vi "UI Build Holding Reg CMD.vi"(8 "error in (no error)":errorcluster, 9 "Message Data":variant, 11 "DAQ DO ON-OFF":refnum<queue>) -> (0 "error out":errorcluster, 1 "CMD Data":variant, 3 "CMD Queue out":refnum<queue>)   [LabVIEW 2020]
uses:
  support/Message Queue/Message Cluster.ctl
  support/Message Queue/Message Queue.lvlib
panel:
  in  "Register":T1(ring)
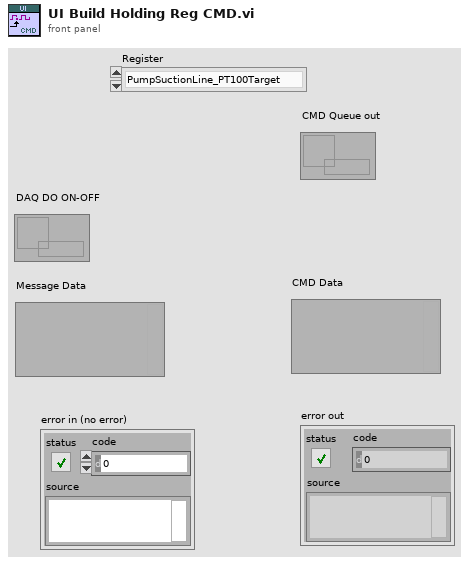
[diagram p1: front panel]
types:
  T1 = enum16{"PumpSuctionLine_PT100Target", "PumpSuctionLine_PT100LimitMin", "PumpSuctionLine_PT100LimitMax", "PumpMainLine_PressureTarget", "PumpMainLine_PressureTargetMin", "PumpMainLine_PressureTargetMax", "RPMTarget", "RPMTargetMax", "RPMTargetMin", "PumpSuctionLine_PressureTarget", "PumpSuctionLine_PressureTargetMin", "PumpSuctionLine_PressureTargetMax", "PumpMainLine_MaxPressureLimit", "PumpSuctionLine_MaxPressureLimit", "PumpSuctionLine_MinPressureLimit", "PumpDrainLine_MaxPressureLimit", "PumpReplenishmentLine_MinPressureLimit", "DrainMinusSuctionPressureLimit", "Torque_MaxLimit", "SectorNumber", "RowNumber", "ProcedureNumber", "ResetControl", "DigitalControl", "CommNumber", "ProcessTimerTarget"}
  T2 = cluster{"Register":enum16{"PumpSuctionLine_PT100Target", "PumpSuctionLine_PT100LimitMin", "PumpSuctionLine_PT100LimitMax", "PumpMainLine_PressureTarget", "PumpMainLine_PressureTargetMin", "PumpMainLine_PressureTargetMax", "RPMTarget", "RPMTargetMax", "RPMTargetMin", "PumpSuctionLine_PressureTarget", "PumpSuctionLine_PressureTargetMin", "PumpSuctionLine_PressureTargetMax", "PumpMainLine_MaxPressureLimit", "PumpSuctionLine_MaxPressureLimit", "PumpSuctionLine_MinPressureLimit", "PumpDrainLine_MaxPressureLimit", "PumpReplenishmentLine_MinPressureLimit", "DrainMinusSuctionPressureLimit", "Torque_MaxLimit", "SectorNumber", "RowNumber", "ProcedureNumber", "ResetControl", "DigitalControl", "CommNumber", "ProcessTimerTarget"}, "value":u16}
  T3 = typedef "Test Names.ctl" = u16
  T4 = cluster{"Register":enum16{"PumpSuctionLine_PT100Target", "PumpSuctionLine_PT100LimitMin", "PumpSuctionLine_PT100LimitMax", "PumpMainLine_PressureTarget", "PumpMainLine_PressureTargetMin", "PumpMainLine_PressureTargetMax", "RPMTarget", "RPMTargetMax", "RPMTargetMin", "PumpSuctionLine_PressureTarget", "PumpSuctionLine_PressureTargetMin", "PumpSuctionLine_PressureTargetMax", "PumpMainLine_MaxPressureLimit", "PumpSuctionLine_MaxPressureLimit", "PumpSuctionLine_MinPressureLimit", "PumpDrainLine_MaxPressureLimit", "PumpReplenishmentLine_MinPressureLimit", "DrainMinusSuctionPressureLimit", "Torque_MaxLimit", "SectorNumber", "RowNumber", "ProcedureNumber", "ResetControl", "DigitalControl", "CommNumber", "ProcessTimerTarget"}, "value":u16}[]
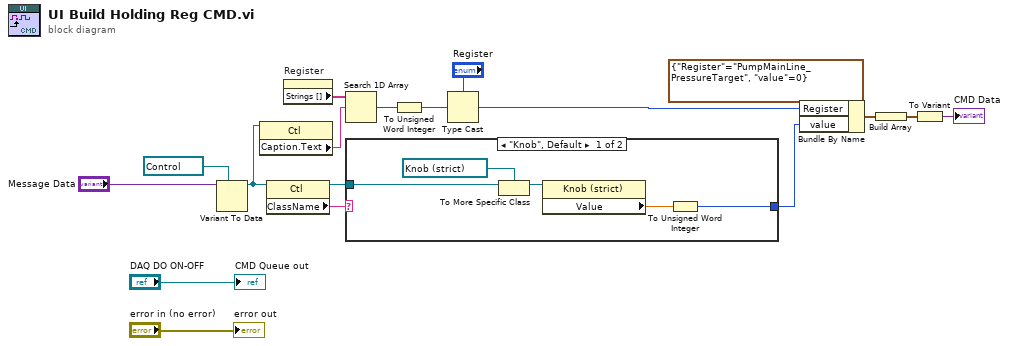
[diagram p0: block diagram]
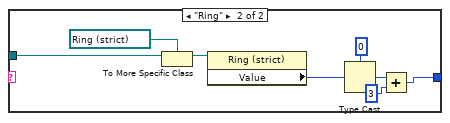
[diagram p2: hidden frame]
diagram:
  n1 = Variant To Data(type=refnum<vi> refnum ("CtlRef"), Variant="Message Data") -> (data=w2:refnum<vi>)  [unwired: 1 in, 1 out]
  n2 = property class="Ctl"(reference=w2) -> ("Caption.Text"=w14:string)  [unwired: 1 in, 2 out]
  n3 = property class="Ctl"(reference=w2) -> (reference out=w3:refnum<vi>, "ClassName"=w4:string)  [unwired: 1 in, 1 out]
  n4 = property on="Register" class="Enum (strict)"() -> ("Strings []"=w13:string[])  [unwired: 2 in, 2 out]
  n5 = Search 1D Array(1D array=w13, element=w14) -> (index of element=w11:i32)  [unwired: 1 in]
  n6 = case shown="\"Knob\", Default" w4 {
    tunnel: w3 -> [w23 w31]
    tunnel: [w19 w25] -> w1
    frame "Knob", Default {
      n7 = To More Specific Class(target class=refnum<vi> refnum ("Manual Air Pressure Control"), reference=w23) -> (specific class reference=w21:refnum<vi>)  [unwired: 1 in, 1 out]
      n8 = property class="Knob (strict)"(reference=w21) -> ("Value"=w20:dbl)  [unwired: 1 in, 2 out]
      n9 = To Unsigned Word Integer(number=w20) -> (unsigned 16bit integer=w19:u16)
    }
    frame "Ring" {
      n10 = To More Specific Class(target class=refnum<vi> refnum ("Current Test"), reference=w31) -> (specific class reference=w30:refnum<vi>)  [unwired: 1 in, 1 out]
      n11 = property class="Ring (strict)"(reference=w30) -> ("Value"=w28:T3)  [unwired: 1 in, 2 out]
      n12 = Type Cast(type=u16 0, x=w28) -> (*(type *) &x=w26:u16)
      n13 = Add(x=w26, y=u16 3) -> (x+y=w25:u16)
    }
  }
  n14 = To Unsigned Word Integer(number=w11) -> (unsigned 16bit integer=w12:u16)
  n15 = Type Cast(type="Register", x=w12) -> (*(type *) &x=w17:T1)
  n16 = Bundle By Name(cluster=T2 {"Register"=enum."PumpMainLine_PressureTarget", "value"=0}, "Register"=w17, "value"=w1) -> (w18:T2)
  n17 = Build Array(w18) -> (w5:T4)
  n18 = To Variant(anything=w5) -> (Variant=→"CMD Data":variant)
  "CMD Queue out" <- "DAQ DO ON-OFF"
  "error out" <- "error in (no error)"
